vi "issueCommandStart.vi"(8 "error in (no error)":errorcluster, 10 "String":string, 11 "SALCommunicatorTC in":refnum<class "SALCommunicatorTC.lvclass">) -> (0 "error out":errorcluster, 3 "SALCommunicatorTC out":refnum<class "SALCommunicatorTC.lvclass">)   [LabVIEW 2016, in "SALCommunicatorTC.lvclass"]
uses:
  SALCommunicatorTC.lvclass
  ts_sallv_exa/DataTypes/command_start.ctl
  ts_sallv_exa/SALLV_EXA.lvlib
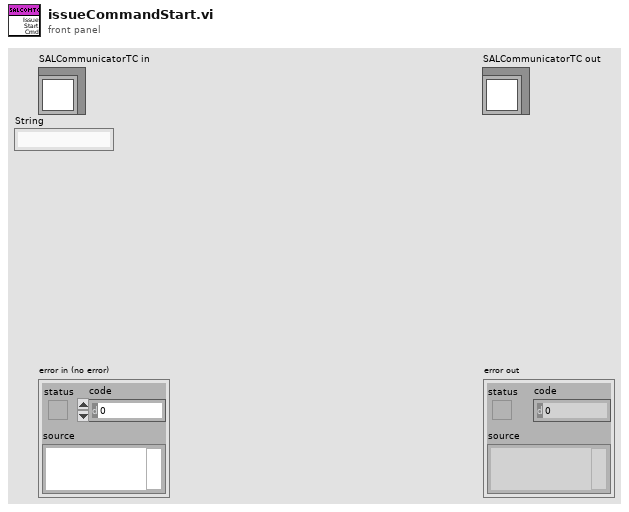
[diagram p1: front panel]
types:
  T1 = typedef "SALLV_EXA.lvlib/command_start.ctl" = cluster{"configuration":string}
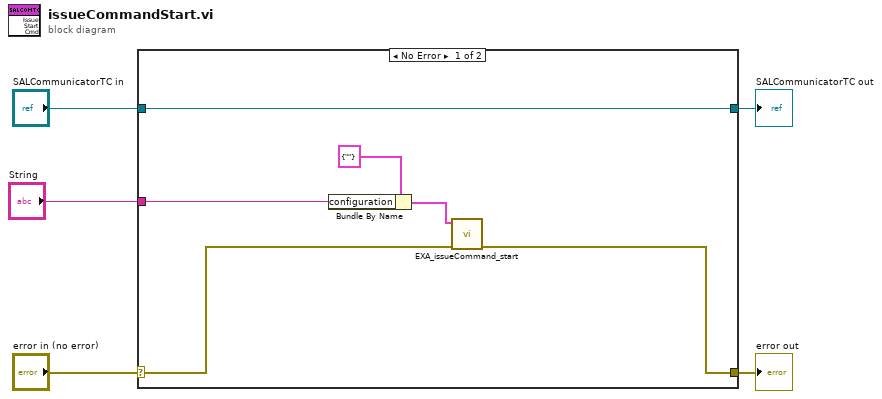
[diagram p0: block diagram]
diagram:
  n1 = case shown="No Error" "error in (no error)" {
    selector: "error in (no error)" -> [w10 w13]
    tunnel: [w9 w13] -> w4
    tunnel: [w11 w12] -> w2
    tunnel: "SALCommunicatorTC in" -> [w11 w12]
    tunnel: "String" -> [w7 _]
    frame No Error {
      n2 = Bundle By Name(cluster=T1 {"configuration"=""} ("command_start_Ctl"), "configuration"=w7) -> (w6:T1)
      n3 = call "EXA_issueCommand_start.vi"("error in (no error)"=w10, "command_start_Ctl"=w6) -> ("error out"=w9:errorcluster)  [unwired: 7 in, 2 out]
    }
    frame Error {
    }
  }
  "error out" <- w4
  "SALCommunicatorTC out" <- w2
